vi "extract indicator data.vi"(9 "dataProcessor":T2, 10 "data in":variant, 11 "Queues in":T5) -> (1 "dataProcessor out":T2, 3 "data out":dbl[][](array[numeric]))   [LabVIEW 2018]
uses:
  type defs/Queues.ctl
  type defs/data processor data.ctl
  type defs/channelLimitControl.ctl
  type defs/limitActions.ctl
  type defs/liveArray.ctl
  supporting VIs/polymorphic VIs/enqueue for user interface.vi
  type defs/localSharedVariables.lvlib
panel:
  out "output cluster":T1
  out "Table Control":string[][](table)
  in  "show values":bool
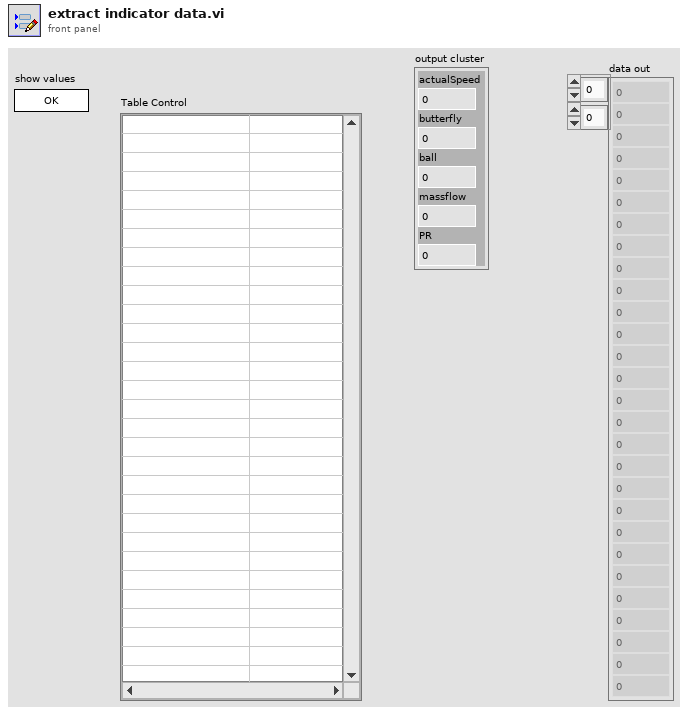
[diagram p1: front panel]
types:
  T1 = cluster{"actualSpeed":dbl, "butterfly":dbl, "ball":dbl, "massflow":dbl, "PR":dbl}
  T2 = typedef "data processor data.ctl" = cluster{"params":cluster{"controlFeedback":cluster{"butterflyValue":u16, "ballValue":u16, "massflow":u16, "pressureRatio":u16, "compSpeed":u16}, "DAQrate":enum16{"50 kHz", "25 kHz", "16.6 kHz", "12.5 kHz", "10 kHz", "8.33 kHz", "7.14 kHz", "6.25 kHz", "5.55 kHz", "5 kHz"}, "safetyChannels":cluster{"oilP":u16, "airP":u16, "water":u16, "channelLimit":T3[]}, "channelConfigPath":path}, "vars":cluster{"controlFeedback":cluster{"butterflyValue":u16, "ballValue":u16, "massflow":u16, "pressureRatio":u16, "compSpeed":u16}, "activeChannelNames":string[], "activeChannelUnits":string[], "offset trigger":bool, "offsets":dbl[], "activeChannelLimitIndex":u16[], "liveData":bool}}
  T3 = typedef "channelLimitControl.ctl" = cluster{"channelID":u16, "Enabled":bool, "warnValue":dbl, "limitValue":dbl, "Invert":bool, "limitAction":T4}
  T4 = typedef "limitActions.ctl" = enum16{"stop", "shutdown", "ignore"}
  T5 = typedef "Queues.ctl" = cluster{"messageHandler":refnum<queue>, "comms":refnum<queue>, "dataStream":refnum<queue>, "dataProcessor":refnum<queue>, "fileIO":refnum<queue>, "userInterface":refnum<queue>, "errors":refnum<queue>, "customCompressor":refnum<queue>}
  T6 = typedef "localSharedVariables.lvlib/liveArray.ctl" = cluster{"ID":u32, "data":dbl[][], "updateRate":u32}
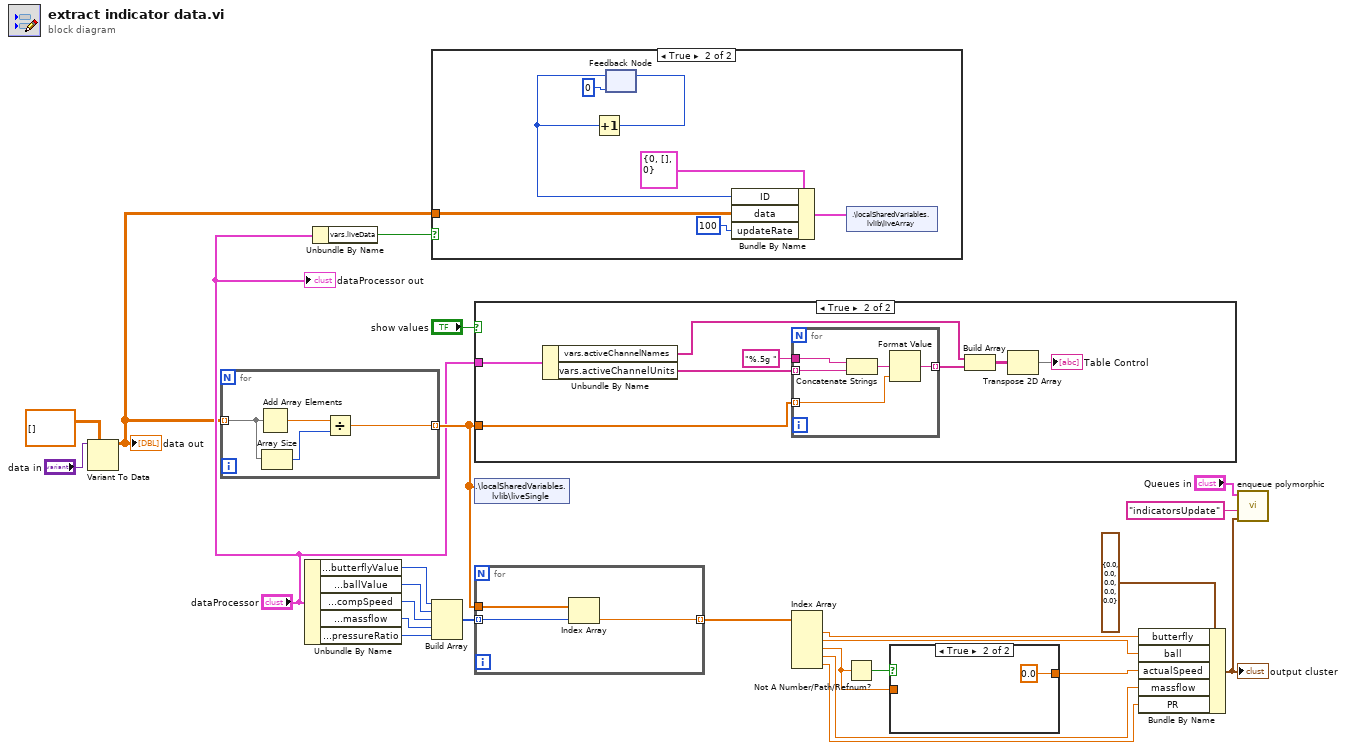
[diagram p0: block diagram]
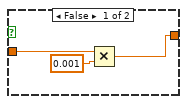
[diagram p3: hidden frame]
diagram:
  n1 = Variant To Data(type=dbl[][] [], Variant="data in") -> (data=w1:dbl[][])  [unwired: 1 in, 1 out]
  "data out" <- w1
  n2 = for {
    tunnel: w1 -> [w27] mode=indexing
    tunnel: [w26] -> w9 mode=indexing
    n3 = Add Array Elements(numeric array=w27) -> (sum=w29:dbl)
    n4 = Array Size(array=w27) -> (size(s)=w28:i32)
    n5 = Divide(x=w29, y=w28) -> (x/y=w26:dbl)
  }
  n6 = Unbundle By Name("dataProcessor") -> ("vars.controlFeedback.butterflyValue"=w16:u16, "vars.controlFeedback.ballValue"=w15:u16, "vars.controlFeedback.compSpeed"=w8:u16, "vars.controlFeedback.massflow"=w7:u16, "vars.controlFeedback.pressureRatio"=w6:u16)
  n7 = Unbundle By Name("dataProcessor") -> ("vars.liveData"=w2:bool)
  n8 = case shown="True" w2 {
    tunnel: w1 -> [_ w31]
    frame False {
    }
    frame True {
      n9 = feedback #1(u32 0) -> (w32:u32)
      n10 = Increment(x=w32) -> (x+1=w34:u32)
      n11 = feedback-in #1(w34) -> ()
      n12 = Bundle By Name(cluster=T6 {"ID"=0, "data"=[], "updateRate"=0} ("liveArray"), "ID"=w32, "data"=w31, "updateRate"=u32 100) -> (w35:T6)
      n13 = shared-variable ".\\localSharedVariables.lvlib\\liveArray"(w35) -> ()  [unwired: 1 in, 1 out]
    }
  }
  n14 = Build Array(w16, w15, w8, w7, w6) -> (w14:u16[])
  n15 = case shown="True" "show values" {
    tunnel: w9 -> [_ w37]
    tunnel: "dataProcessor" -> [_ w44]
    frame False {
    }
    frame True {
      n16 = Unbundle By Name(w44) -> ("vars.activeChannelNames"=w40:string[], "vars.activeChannelUnits"=w43:string[])
      n17 = for {
        tunnel: w37 -> [w49] mode=indexing
        tunnel: w43 -> [w48] mode=indexing
        tunnel: "%.5g " ("format string") -> [w47]
        tunnel: [w45] -> w41 mode=indexing
        n18 = Concatenate Strings(w47, w48) -> (w46:string)
        n19 = Format Value(format string=w46, value (0)=w49) -> (output string=w45:string)  [unwired: 1 in]
      }
      n20 = Build Array(w40, w41) -> (w39:string[][])
      n21 = Transpose 2D Array(2D array=w39) -> (transposed array=→"Table Control":string[][])
    }
  }
  n22 = shared-variable ".\\localSharedVariables.lvlib\\liveSingle"(w9) -> ()  [unwired: 1 in, 1 out]
  n23 = for {
    tunnel: w9 -> [w52]
    tunnel: w14 -> [w51] mode=indexing
    tunnel: [w50] -> w22 mode=indexing
    n24 = Index Array(array=w52, index=w51) -> (element=w50:dbl)
  }
  n25 = Index Array(array=w22) -> (element #1=w21:dbl, element #2=w20:dbl, element #3=w11:dbl, element #4=w5:dbl, element #5=w4:dbl)  [unwired: 5 in]
  n26 = Not A Number/Path/Refnum?(number/path/refnum=w11) -> (NaN/Path/Refnum?=w10:bool)
  n27 = case shown="True" w10 {
    tunnel: [w55 0.0] -> w12
    tunnel: w11 -> [w53 _]
    frame False {
      n28 = Multiply(x=w53, y=0.001) -> (x*y=w55:dbl)
    }
    frame True {
    }
  }
  n29 = Bundle By Name(cluster=T1 {"actualSpeed"=0.0, "butterfly"=0.0, "ball"=0.0, "massflow"=0.0, "PR"=0.0} ("indicators"), "butterfly"=w21, "ball"=w20, "actualSpeed"=w12, "massflow"=w5, "PR"=w4) -> (w17:T1)
  "output cluster" <- w17
  n30 = call-poly "enqueue polymorphic.vi"("data"=w17, "message"="indicatorsUpdate", "Queues"="Queues in") -> ()  [unwired: 8 in, 1 out]
  "dataProcessor out" <- "dataProcessor"
